vi "VCI_CAN_OBJ_U8ARR_CONVERT.vi"(1 "U8_Arr":u8[](array[numeric])) -> (0 "VCI_CAN_OBJ":T1)   [LabVIEW 2018, in "ControlCan.lvlib"]
uses:
  ControlCan.lvlib
  VCI_CAN_OBJ.ctl
  VCI_CAN_OBJ_1.ctl
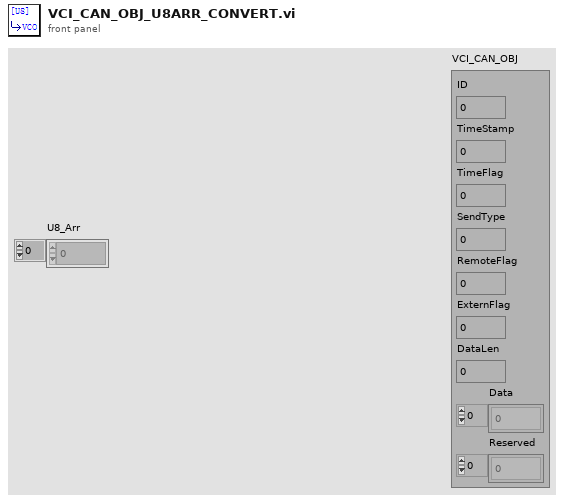
[diagram p1: front panel]
types:
  T1 = typedef "ControlCAN.lvlib/VCI_CAN_OBJ.ctl" = cluster{"ID":u32, "TimeStamp":u32, "TimeFlag":u8, "SendType":u8, "RemoteFlag":u8, "ExternFlag":u8, "DataLen":u8, "Data":u8[], "Reserved":u8[]}
  T2 = typedef "ControlCAN.lvlib/VCI_CAN_OBJ_1.ctl" = cluster{"ID":u32, "TimeStamp":u32, "TimeFlag":u8, "SendType":u8, "RemoteFlag":u8, "ExternFlag":u8, "DataLen":u8, "Data 0":u8, "Data 1":u8, "Data 2":u8, "Data 3":u8, "Data 4":u8, "Data 5":u8, "Data 6":u8, "Data 7":u8, "Reserved 0":u8, "Reserved 1":u8, "Reserved 2":u8}
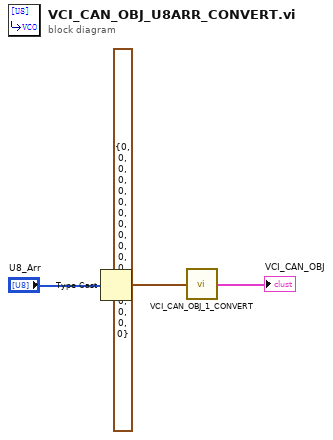
[diagram p0: block diagram]
diagram:
  n1 = Type Cast(type=T2 {"ID"=0, "TimeStamp"=0, "TimeFlag"=0, "SendType"=0, "RemoteFlag"=0, "ExternFlag"=0, "DataLen"=0, "Data 0"=0, "Data 1"=0, "Data 2"=0, "Data 3"=0, "Data 4"=0, "Data 5"=0, "Data 6"=0, "Data 7"=0, "Reserved 0"=0, "Reserved 1"=0, "Reserved 2"=0} ("VCI_CAN_OBJ_1"), x="U8_Arr") -> (*(type *) &x=w2:T2)
  n2 = call "VCI_CAN_OBJ_1_CONVERT.vi"("VCI_CAN_OBJ_1"=w2) -> ("VCI_CAN_OBJ"=→"VCI_CAN_OBJ":T1)
